vi "Set Default Case.vi"(8 "error in (no error)":errorcluster, 10 "Case Index":i32, 11 "Case Structure in":refnum<vi>) -> (0 "error out":errorcluster, 3 "Case Structure out":refnum<vi>)   [LabVIEW 2019, in "gRPC Template Creation Utility.lvlib"]
uses:
  gRPC Template Creation Utility.lvlib
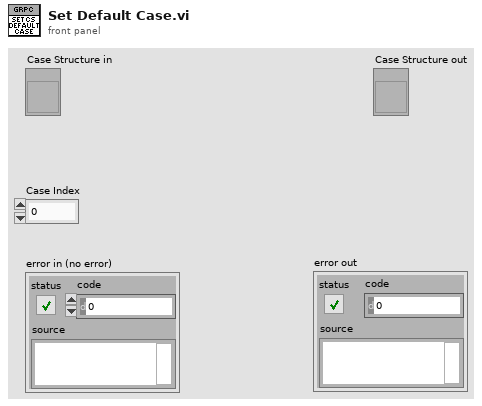
[diagram p1: front panel]
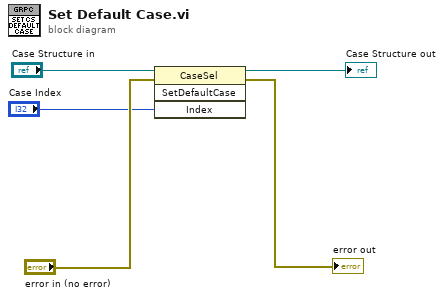
[diagram p0: block diagram]
diagram:
  n1 = invoke class="CaseSel" method="SetDefaultCase"(reference="Case Structure in", error in="error in (no error)", "Index"="Case Index") -> (reference out=→"Case Structure out":refnum<vi>, error out=→"error out":errorcluster)  [unwired: 1 in, 2 out]
